vi "表格数据输入-8.6.vi"(6 "列数?":bool, 8 "行数":u32=1, 9 "列数":u32=1, 10 "字符串数组":string[](array[string])=["300", "250", "120"], 11 "表格引用":refnum<vi>) -> ()   [LabVIEW 2013]
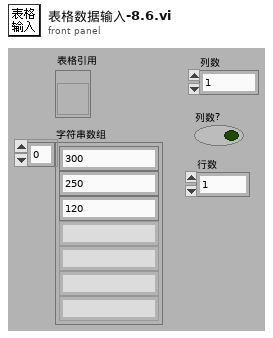
[diagram p1: front panel]
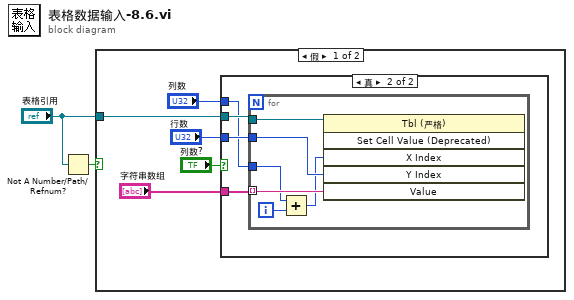
[diagram p0: block diagram]
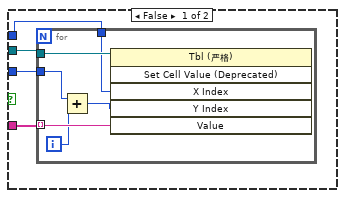
[diagram p2: hidden frame]
diagram:
  n1 = Not A Number/Path/Refnum?(number/path/refnum="表格引用") -> (NaN/Path/Refnum?=w2:bool)
  n2 = case shown="假" w2 {
    tunnel: "表格引用" -> [w6 _]
    frame False {
      n3 = case shown="真" "列数?" {
        tunnel: "字符串数组" -> [w11 w21]
        tunnel: w6 -> [w10 w20]
        tunnel: "行数" -> [w9 w19]
        tunnel: "列数" -> [w8 w18]
        frame False {
          n4 = for {
            tunnel: w10 -> [w17]
            tunnel: w11 -> [w16] mode=indexing
            tunnel: w9 -> [w13]
            tunnel: w8 -> [w12]
            i -> [w15]
            n5 = Add(x=w13, y=w15) -> (x+y=w14:u32)
            n6 = invoke class="Tbl (严格)" method="Set Cell Value (Deprecated)"(reference=w17, "X Index"=w12, "Y Index"=w14, "Value"=w16) -> ()  [unwired: 2 in, 6 out]
          }
        }
        frame True {
          n7 = for {
            tunnel: w20 -> [w27]
            tunnel: w21 -> [w26] mode=indexing
            tunnel: w19 -> [w24]
            tunnel: w18 -> [w22]
            i -> [w25]
            n8 = Add(x=w22, y=w25) -> (x+y=w23:u32)
            n9 = invoke class="Tbl (严格)" method="Set Cell Value (Deprecated)"(reference=w27, "X Index"=w23, "Y Index"=w24, "Value"=w26) -> ()  [unwired: 2 in, 6 out]
          }
        }
      }
    }
    frame True {
    }
  }
